vi "re_LuaVIEW Execute Iteration.vi"(5 "LuaVIEW reference in":T1, 11 "init or indexed function error":errorcluster) -> (4 "last?":bool, 6 "LuaVIEW reference out":T1, 8 "function index":i32, 15 "final error":errorcluster)   [LabVIEW 2013]
doc: "Execute compiled script(s) for a single \"resume\" iteration and return to LabVIEW when the last script completes, a LabVIEW-side call is made, a yield is performed, an error occurs, and so on. Iterating over resumptions allows LabVIEW-side stuff to be interspersed with virtual machine execution. Any custom LabVIEW-side stuff, such as indexed functions or execution management must be implemented as part of the loop inside which this VI is called."
uses:
  typedefs/t_LuaVIEW Reference.ctl
  typedefs/et_LuaVIEW CIN Actions.ctl
  typedefs/t_LuaVIEW CIN Spinlocked Actions.ctl
  glb_LuaVIEW Configuration Globals.vi
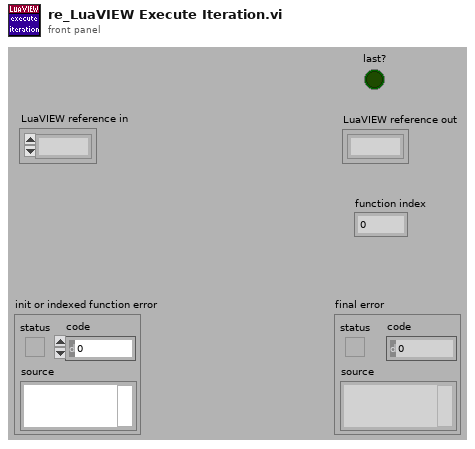
[diagram p1: front panel]
types:
  T1 = typedef "t_LuaVIEW Reference.ctl" = refnum<k1>
  T2 = typedef "et_LuaVIEW CIN Actions.ctl" = enum16{"checksynopsis", "_open", "_registerpublic", "_registerexport", "__never_an_error_result_ns", "luaversion", "cinversion", "_totals", "_taskcount", "pathological", "_unregnextpublic", "registryusecount", "__per_state_actions", "regsetprivate", "regsetindex", "regsetmodule", "_revokeexports", "_usepublic", "prepare", "compile", "execute", "call", "unregstaterefs", "_close", "pullboolean", "pullnumber", "pullI8", "pullU8", "pullI16", "pullU16", "pullI32", "pullU32", "pullobject", "pullrefnum", "pullstring", "pullflat", "pushflat", "pushobject", "getattribute", "setattribute", "stacktostring", "_startyieldtest", "_endyieldtest", "_pollprintbuffer", "__never_an_error_result_ps", "_pollexport", "setclone", "forcecleanup", "gettop", "clearstack", "insert", "pushboolean", "pushnumber", "pushrefnum", "pushstring", "pushnil", "pushvalue", "gettaskref", "settaskref"}
  T3 = typedef "t_LuaVIEW CIN Spinlocked Actions.ctl" = enum16{"totals", "taskcount", "open", "registerpublic", "registerexport", "revokeexports", "unregnextpublic", "usepublic", "pollexport", "close", "startyieldtest", "endyieldtest", "pollprintbuffer"}
  T4 = typedef "et_LuaVIEW CIN Results.ctl" = enum16{"OK", "error", "main", "call", "clonecall", "modulecall", "exportcall", "index", "yield"}
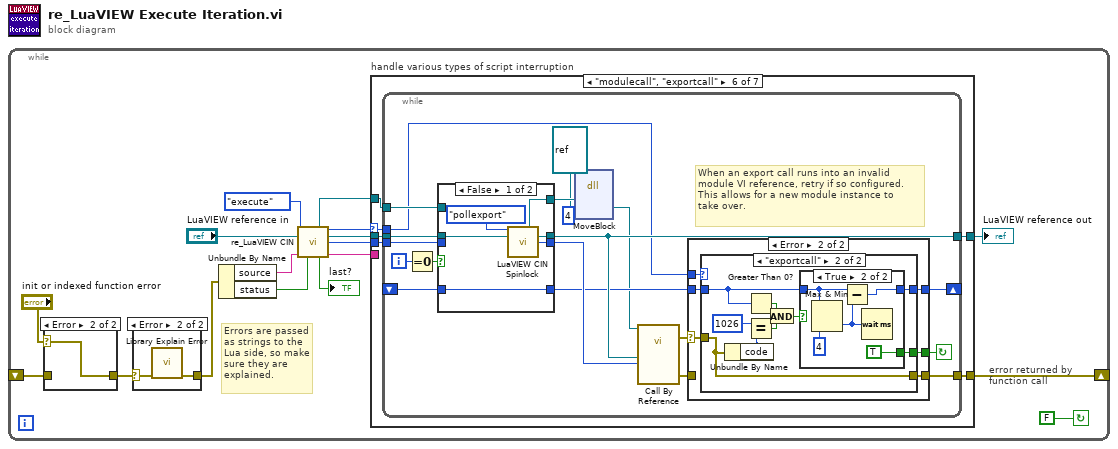
[diagram p0: block diagram]
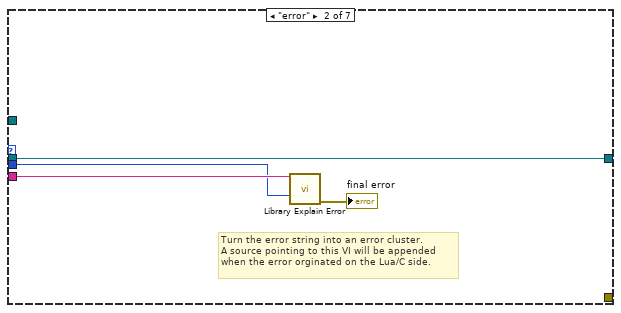
[diagram p5: hidden frame]
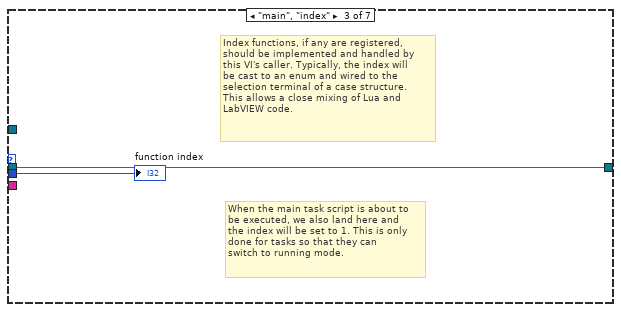
[diagram p6: hidden frame]
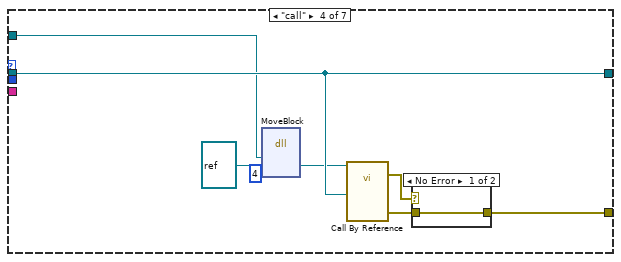
[diagram p7: hidden frame]
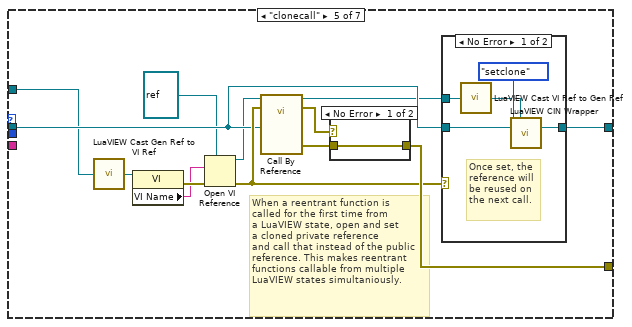
[diagram p9: hidden frame]
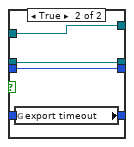
[diagram p12: hidden frame]
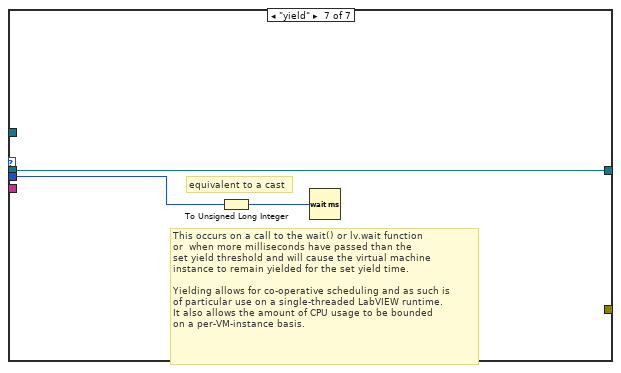
[diagram p16: hidden frame]
diagram:
  n1 = while {
    shift-right: [w8] -> _
    shift-left: _ -> [w6]
    stop <- FALSE continue-if-true
    # "Errors are passed as strings to the Lua side, so make sure they are explained."
    # "error returned by\nfunction call"
    n2 = case shown="Error" "init or indexed function error" {
      selector: "init or indexed function error" -> [_ w22]
      tunnel: w6 -> [w21 _]
      tunnel: [w21 w22] -> w2
      frame No Error {
      }
      frame Error {
      }
    }
    n3 = case shown="Error" w2 {
      selector: w2 -> [w18 w20]
      tunnel: [w18 w19] -> w1
      frame No Error {
      }
      frame Error {
        n4 = call "Library Explain Error.vi"("error in (no error)"=w20) -> ("explained error"=w19:errorcluster)  [unwired: 14 in]
      }
    }
    n5 = Unbundle By Name(w1) -> ("source"=w3:string, "status"=w5:bool)
    n6 = call "re_LuaVIEW CIN.vi"("action"=et_LuaVIEW_CIN_Actions."execute", "LuaVIEW reference in"="LuaVIEW reference in", "string in"=w3, "boolean in"=w5) -> ("refnum out"=w10:refnum<vi>, "result"=w15:T4, "LuaVIEW reference out"=w13:T1, "index out"=w11:i32, "boolean out"=→"last?":bool, "string out"=w12:string)  [unwired: 5 in, 1 out]
    n7 = case "handle various types of script interruption" shown="\"modulecall\", \"exportcall\"" w15 {
      selector: w15 -> [_ _ _ _ _ w61 _]
      tunnel: w13 -> [w23 w27 w29 w36 w45 w65 w123]
      tunnel: [w23 w27 w29 w36 w50 w62 w123] -> w16
      tunnel: w12 -> [_ w26 _ _ _ _ _]
      tunnel: w11 -> [_ w24 w28 _ _ w63 w122]
      tunnel: w10 -> [_ _ _ w32 w42 w66 _]
      tunnel: [_ _ _ w34 w48 w64 _] -> w8
      frame "OK" {
        # "If OK, initial setup, the next compilation, or one of the cleanup functions has completed."
      }
      frame "error" {
        # "Turn the error string into an error cluster.\nA source pointing to this VI will be appended\nwhen the error orginated on the Lua/C side."
        n8 = call "Library Explain Error.vi"("explanation prefix (none)"=w26, "skip levels (0)"=w24) -> ("explained error"=→"final error":errorcluster)  [unwired: 13 in]
      }
      frame "main", "index" {
        # "When the main task script is about to\nbe executed, we also land here and\nthe index will be set to 1. This is only\ndone for tasks so that they can\nswitch to running mode."
        # "Index functions, if any are registered,\nshould be implemented and handled by\nthis VI's caller. Typically, the index will\nbe cast to an enum and wired to the\nselection terminal of a case structure.\nThis allows a close mixing of Lua and\nLabVIEW code."
        "function index" <- w28
      }
      frame "call" {
        n9 = dll-call lib="LabVIEW" fn="MoveBlock"("refnum out"=w32, "function pane"=refnum<vi> refnum, "len"=4) -> ("function pane"=w30:refnum<vi>)  [unwired: 6 in, 2 out]
        n10 = call-by-ref "?"(reference=w30, "LuaVIEW reference"=w36) -> (error out=w37:errorcluster, 15:"error out"=w35:errorcluster)  [unwired: 15 in, 1 out]
        n11 = case shown="No Error" w37 {
          selector: w37 -> [_ w39]
          tunnel: [w38 w39] -> w34
          tunnel: w35 -> [w38 _]
          frame No Error {
          }
          frame Error {
          }
        }
      }
      frame "clonecall" {
        # "When a reentrant function is\ncalled for the first time from\na LuaVIEW state, open and set\na cloned private reference\nand call that instead of the public\nreference. This makes reentrant\nfunctions callable from multiple\nLuaVIEW states simultaniously."
        n12 = call "LuaVIEW Cast Gen Ref to VI Ref.vi"("refnum in"=w42) -> ("refnum out"=w43:refnum<vi>)  [unwired: 14 in]
        n13 = property class="VI"(reference=w43) -> (error out=w51:errorcluster, "VI Name"=w46:string)  [unwired: 1 in, 1 out]
        n14 = Open VI Reference(type specifier VI Refnum (for type only)=refnum<vi> refnum ("function pane"), vi path=w46, error in (no error)=w51) -> (vi reference=w44:refnum<vi>, error out=w47:errorcluster)  [unwired: 3 in]
        n15 = call-by-ref "?"(reference=w44, error in=w47, "LuaVIEW reference"=w45) -> (reference out=w41:refnum<vi>, error out=w52:errorcluster, 15:"error out"=w49:errorcluster)  [unwired: 14 in]
        n16 = case shown="No Error" w52 {
          selector: w52 -> [_ w60]
          tunnel: [w59 w60] -> w48
          tunnel: w49 -> [w59 _]
          frame No Error {
          }
          frame Error {
          }
        }
        n17 = case shown="No Error" w47 {
          tunnel: w45 -> [w56 w58]
          tunnel: [w55 w58] -> w50
          tunnel: w41 -> [w54 _]
          frame No Error {
            # "Once set, the\nreference will\nbe reused on\nthe next call."
            n18 = call "LuaVIEW Cast VI Ref to Gen Ref.vi"("refnum in"=w54) -> ("refnum out"=w53:refnum<vi>)  [unwired: 14 in]
            n19 = call "LuaVIEW CIN Wrapper.vi"("action"=et_LuaVIEW_CIN_Actions."setclone", "refnum in"=w53, "LuaVIEW reference in"=w56) -> ("LuaVIEW reference out"=w55:T1)  [unwired: 12 in]
          }
          frame Error {
          }
        }
      }
      frame "modulecall", "exportcall" {
        n20 = while {
          tunnel: w66 -> [w77]
          tunnel: w65 -> [w81]
          tunnel: [w83] -> w64
          tunnel: w63 -> [w79]
          tunnel: [w80] -> w62
          shift-right: [w72] -> _
          shift-left: _ -> [w75]
          tunnel: w61 -> [w74]
          i -> [w82]
          stop <- w71 continue-if-true
          # "When an export call runs into an invalid\nmodule VI reference, retry if so configured.\nThis allows for a new module instance to\ntake over."
          n21 = Equal To 0?(x=w82) -> (x = 0?=w76:bool)
          n22 = case shown="False" w76 {
            tunnel: w81 -> [w91 w94]
            tunnel: [w90 w94] -> w80
            tunnel: [w89 w93] -> w69
            tunnel: w79 -> [_ w95]
            tunnel: [w88 w95] -> w78
            tunnel: w77 -> [_ w93]
            tunnel: w75 -> [w86 _]
            tunnel: [w86 w92] -> w73
            frame False {
              n23 = call "LuaVIEW CIN Spinlock.vi"("action"=t_LuaVIEW_CIN_Spinlocked_Actions."pollexport", "LuaVIEW reference in"=w91) -> ("refnum out"=w89:refnum<vi>, "LuaVIEW reference out"=w90:T1, "index out"=w88:i32)  [unwired: 7 in, 4 out]
            }
            frame True {
              n24 = global read "glb_LuaVIEW Configuration Globals.vi" "export timeout"() -> (w92:u32)
            }
          }
          n25 = dll-call lib="LabVIEW" fn="MoveBlock"("refnum out"=w69, "module pane"=refnum<vi> refnum, "len"=4) -> ("module pane"=w68:refnum<vi>)  [unwired: 6 in, 2 out]
          n26 = call-by-ref "?"(reference=w68, "LuaVIEW reference"=w80, "function index"=w78) -> (error out=w85:errorcluster, 15:"error out"=w84:errorcluster)  [unwired: 14 in, 1 out]
          n27 = case shown="Error" w85 {
            selector: w85 -> [_ w103]
            tunnel: [w97 w102] -> w83
            tunnel: w84 -> [w97 _]
            tunnel: w74 -> [_ w101]
            tunnel: w73 -> [w96 w100]
            tunnel: [w96 w99] -> w72
            tunnel: [_ w98] -> w71
            frame No Error {
            }
            frame Error {
              n28 = case shown="\"exportcall\"" w101 {
                tunnel: w103 -> [w105 w112]
                tunnel: [w105 w112] -> w102
                tunnel: [w104 w107] -> w99
                tunnel: w100 -> [w104 w108]
                tunnel: [_ w106] -> w98
                frame Default {
                }
                frame "exportcall" {
                  n29 = Unbundle By Name(w112) -> ("code"=w114:i32)
                  n30 = Greater Than 0?(x=w108) -> (x > 0?=w111:bool)
                  n31 = Equal?(x=1026, y=w114) -> (x = y?=w110:bool)
                  n32 = And(x=w111, y=w110) -> (x .and. y?=w109:bool)
                  n33 = case shown="True" w109 {
                    tunnel: w108 -> [w115 w119]
                    tunnel: [w115 w117] -> w107
                    tunnel: [_ TRUE] -> w106
                    frame False {
                    }
                    frame True {
                      n34 = Max & Min(x=w119, y=u32 4 ("export timeout")) -> (min(x,y)=w118:u32)  [unwired: 1 out]
                      n35 = Subtract(x=w119, y=w118) -> (x-y=w117:u32)
                      n36 = Wait (ms)(milliseconds to wait=w118) -> ()  [unwired: 1 out]
                    }
                  }
                }
              }
            }
          }
        }
      }
      frame "yield" {
        # "equivalent to a cast"
        # "This occurs on a call to the wait() or lv.wait function\nor  when more milliseconds have passed than the\nset yield threshold and will cause the virtual machine\ninstance to remain yielded for the set yield time.\n\nYielding allows for co-operative scheduling and as such is\nof particular use on a single-threaded LabVIEW runtime.\nIt also allows the amount of CPU usage to be bounded\non a per-VM-instance basis."
        n37 = To Unsigned Long Integer(number=w122) -> (unsigned 32bit integer=w121:u32)
        n38 = Wait (ms)(milliseconds to wait=w121) -> ()  [unwired: 1 out]
      }
    }
    "LuaVIEW reference out" <- w16
  }
